vi "Check-out.vi"(0 "Guest Manager Model in":refnum<class "Guest Manager Model.lvclass">, 5 "Room No":string, 11 "error in (no error)":errorcluster) -> (4 "Guest Manager Model out":refnum<class "Guest Manager Model.lvclass">, 15 "error out":errorcluster)   [LabVIEW 2023, in "Guest Manager Model.lvlib" / "Guest Manager Model.lvclass"]
uses:
  Guest Manager Model.lvclass
  C:/Program Files/National Instruments/LabVIEW 2023/vi.lib/ActorFramework/Actor/Actor.lvclass
  <vilib>/ActorFramework/Actor/Actor.lvclass/Actor.ctl
  Interfaces/Incoming Rooms Manager Model Interface Messages/Check Guest History Msg/Check Guest History Msg.lvclass/Check Guest History Msg.ctl
  <vilib>/ActorFramework/Message Enqueuer/Message Enqueuer.lvclass/Message Enqueuer.ctl
  <vilib>/ActorFramework/Message Enqueuer/Enqueue.vi
  Interfaces/Incoming Rooms Manager Model Interface Messages/Check Guest History Msg/Check Guest History Msg.lvclass
  C:/Program Files/National Instruments/LabVIEW 2023/vi.lib/ActorFramework/Message/Message.lvclass
  <vilib>/ActorFramework/Message Priority Queue/Priority Enqueue.vi
  Guest Manager Model.lvclass/Guest Manager Model.ctl
  <vilib>/ActorFramework/Actor/Actor.lvclass
  Interfaces/Incoming Rooms Manager Model Interface Messages/Check-Out Msg/Check-Out Msg.lvclass
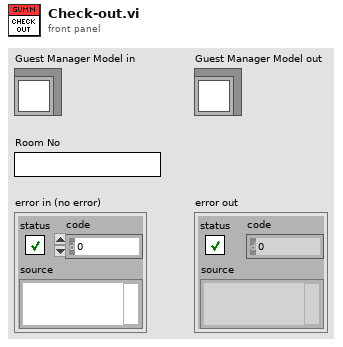
[diagram p1: front panel]
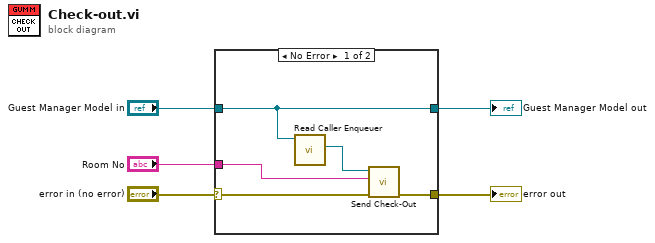
[diagram p0: block diagram]
diagram:
  n1 = case shown="No Error" "error in (no error)" {
    selector: "error in (no error)" -> [w10 w12]
    tunnel: [w9 w12] -> w4
    tunnel: [w8 w11] -> w2
    tunnel: "Guest Manager Model in" -> [w8 w11]
    tunnel: "Room No" -> [w6 _]
    frame No Error {
      n2 = call <vilib>:"Read Caller Enqueuer.vi"("Actor"=w8) -> ("Caller Enqueuer"=w7:refnum<class "Message Enqueuer.lvclass">)  [unwired: 10 in]
      n3 = call "Send Check-Out.vi"("error in (no error)"=w10, "Room No"=w6, "Message Enqueuer"=w7) -> ("error out"=w9:errorcluster)  [unwired: 7 in, 1 out]
    }
    frame Error {
    }
  }
  "error out" <- w4
  "Guest Manager Model out" <- w2
